vi "AudioTest.Get PC Audio Device List.vi"() -> (2 "Output Devices":string[](array[string]), 3 "Input Devices":string[](array[string]))   [LabVIEW 2018]
panel:
  out "Number of Output Devices":i32
  out "Number of Input Devices":i32
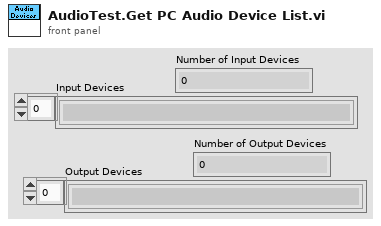
[diagram p1: front panel]
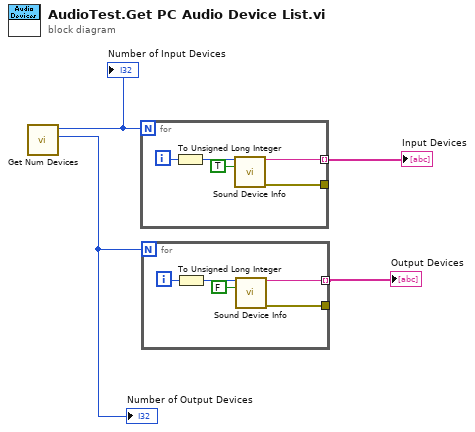
[diagram p0: block diagram]
diagram:
  n1 = call <vilib>:"Get Num Devices.vi"() -> ("Number of Output Devices"=w2:i32, "Number of Input Devices"=w4:i32)  [unwired: 9 in, 1 out]
  "Number of Input Devices" <- w4
  "Number of Output Devices" <- w2
  n2 = for {
    N: w4 -> [_]
    tunnel: [w7] -> w3 mode=indexing
    tunnel: [w6] -> _
    i -> [w8]
    n3 = To Unsigned Long Integer(number=w8) -> (unsigned 32bit integer=w9:u32)
    n4 = call <vilib>:"Sound Device Info.vi"("device"=w9, "isInput?"=TRUE) -> ("Device Name"=w7:string, "error out"=w6:errorcluster)  [unwired: 11 in, 1 out]
  }
  "Input Devices" <- w3
  n5 = for {
    N: w2 -> [_]
    tunnel: [w12] -> w1 mode=indexing
    tunnel: [w11] -> _
    i -> [w13]
    n6 = To Unsigned Long Integer(number=w13) -> (unsigned 32bit integer=w14:u32)
    n7 = call <vilib>:"Sound Device Info.vi"("device"=w14, "isInput?"=FALSE) -> ("Device Name"=w12:string, "error out"=w11:errorcluster)  [unwired: 11 in, 1 out]
  }
  "Output Devices" <- w1
